vi "Right Execute Motion Profile.vi"(0 "Motor Name":string, 5 "Time Conversion Factor":dbl=0.48, 7 "Linear Conversion Factor":dbl, 9 "Motion Profile Array":dbl[][](array[numeric]), 11 "PIDF Profile Slot Select":u8) -> (4 "Complete":bool, 6 "Motion Profiler Data Out":T1)   [LabVIEW 2016]
uses:
  <vilib>/Rock Robotics/WPI/ThirdParty/CanMotor/TalonSRX/WPI_CANTalonSRX_APIControlMode.ctl
  <vilib>/Rock Robotics/WPI/ThirdParty/CanMotor/TalonSRX/WPI_CANTalonSRX_MotionProfileTrajectoryPt.ctl
  Global Variables/Drive Path Logging Data.vi
panel:
  in  "Motion Profiler Data":T1
  out "Execute Loop Index":i32
  out "Execute Is Last":bool
  out "Mot Prof Active Is Last":bool
  out "Waveform Chart":T2(graph)
  out "Mot Prof Active Is Under Run":bool
  out "Mot Prof Active Is Valid":bool
  out "Mot Prof Buffer Is Full":bool
  out "Mot Prof NextID":i32
  out "Mot Prof Count":i32
  out "Mot Prof Output Enable":i32
  out "Total Points in File":i32
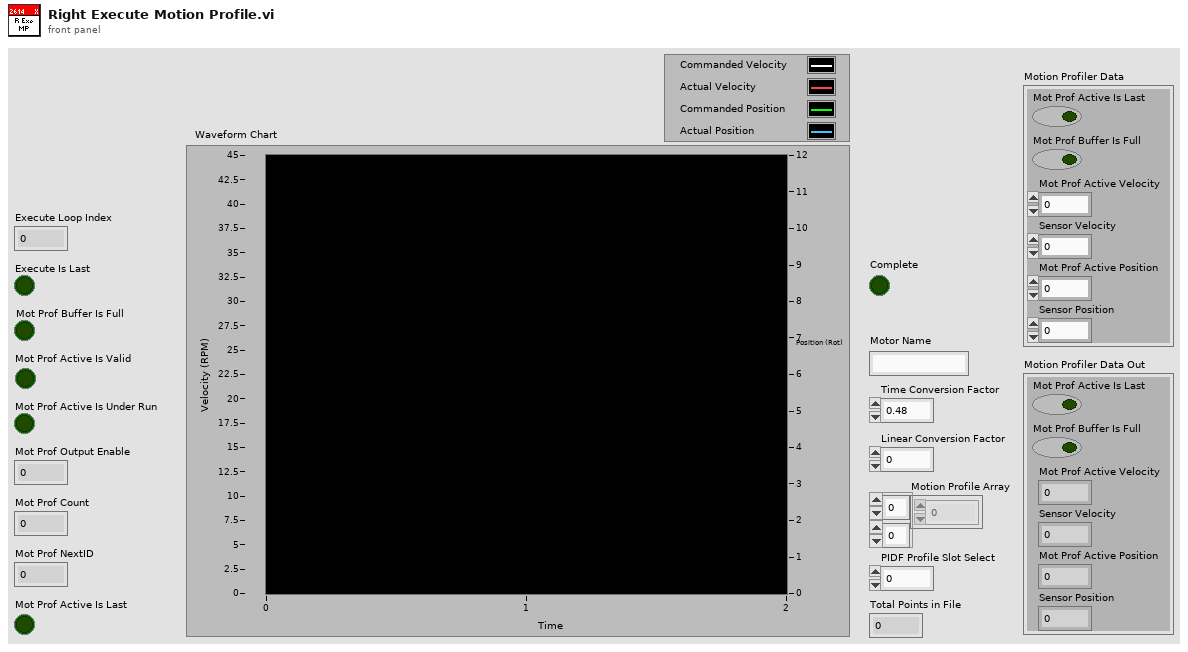
[diagram p1: front panel]
types:
  T1 = cluster{"Mot Prof Active Is Last":bool, "Mot Prof Buffer Is Full":bool, "Mot Prof Active Velocity":dbl, "Sensor Velocity":dbl, "Mot Prof Active Position":dbl, "Sensor Position":dbl}
  T2 = cluster{"Mot Prof Active Velocity":dbl, "Sensor Velocity":dbl, "Mot Prof Active Position":dbl, "Sensor Position":dbl}
  T3 = typedef "WPI_MotorControlDeviceRef.ctl" = cluster{"DeviceStatus":errorcluster, "Type":T4, "PWM":cluster{"PWM Channel":T5, "DeadBand":T6}, "CAN":cluster{"Device Number":u8, "SetOutput VI Ref":variant, "GetOutput VI Ref":variant, "Enable VI Ref":variant, "Disable VI Ref":variant, "Data":variant}, "Invert":bool}
  T4 = typedef "WPI_MotorControlType.ctl" = enum16{"PWM", "CAN"}
  T5 = typedef "FPGA_DIOPWMChannel.ctl" = enum8{"PWM 0", "PWM 1", "PWM 2", "PWM 3", "PWM 4", "PWM 5", "PWM 6", "PWM 7", "PWM 8", "PWM 9", "PWM MXP 0", "PWM MXP 1", "PWM MXP 2", "PWM MXP 3", "PWM MXP 4", "PWM MXP 5", "PWM MXP 6", "PWM MXP 7", "PWM MXP 8", "PWM MXP 9", "Invalid"}
  T6 = typedef "WPI_PWMDeadband.ctl" = cluster{"Name":string, "maxPositivePwm":i32, "minPositivePwm":i32, "centerPwm":i32, "maxNegativePwm":i32, "minNegativePwm":i32, "angularRange":u16}
  T7 = typedef "WPI_CANTalonSRX_APIControlMode.ctl" = enum8{"Percent VBus", "Speed", "Position", "Slave", "Unchanged / Invalid", "Voltage Compensation", "Current", "Motion Profile", "Motion Magic"}
  T8 = typedef "WPI_CANTalonSRX_MotionProfileTrajectoryPt.ctl" = cluster{"Duration Ms":u8, "Velocity":dbl, "Position":dbl, "Profile Slot Select":u8, "Is Last":bool, "Velocity Only":bool, "Zero Position":bool, "Compress Code":u8, "Same Velocity":i32, "Delta Position":i32, "Count":u8}
  T9 = typedef "WPI_CANTalonSRX_GlobalStatus.ctl" = cluster{"Applied Throttle":dbl, "Module Enabled":bool, "CAN Error":errorcluster, "Closed Loop Error":dbl, "Forward Limit Switch Closed":bool, "Reverse Limit Switch Closed":bool, "Sensor Position":dbl, "Sensor Velocity":dbl, "Current":dbl, "Sticky Fault - Over Temp":bool, "Sticky Fault - Under Voltage":bool, "Sticky Fault - Forward Limit":bool, "Sticky Fault - Reverse Limit":bool, "Sticky Fault - Forward Soft Limit":bool, "Sticky Fault - Reverse Soft Limit":bool, "Brake is Enabled":bool, "Encoder Position":dbl, "Encoder Velocity":dbl, "Encoder Index Count":dbl, "Encoder A Pin State":bool, "Encoder B Pin State":bool, "Encoder Index Pin State":bool, "Analog In":dbl, "Analog In Velocity":dbl, "Temperature (C)":dbl, "Battery Voltage":dbl, "Control 5 Is Supported":bool, "Current Profile Slot Select":dbl, "Pos Div 8":bool, "Vel Div 4":bool, "Pulse Width Position":i32, "Pulse Width Velocity":i32, "Pulse Width Rise To Rise (us)":i32, "Pulse Width Rise To Fall (us)":i32, "Mot Prof Active Is Under Run":bool, "Mot Prof Active Has Under Run":bool, "Mot Prof Active Is Last":bool, "Mot Prof Active Velocity Only":bool, "Mot Prof Active Is Valid":bool, "Mot Prof Buffer Is Full":bool, "Mot Prof Active Profile Slot Select":i32, "Mot Prof NextID":i32, "Mot Prof Count":i32, "Mot Prof Active Velocity":dbl, "Mot Prof Active Position":dbl, "Mot Prof Output Enable":i32, "UsageFrame":u32, "Motion Magic Active Trajectory":cluster{"Velocity":dbl, "Position":dbl}}
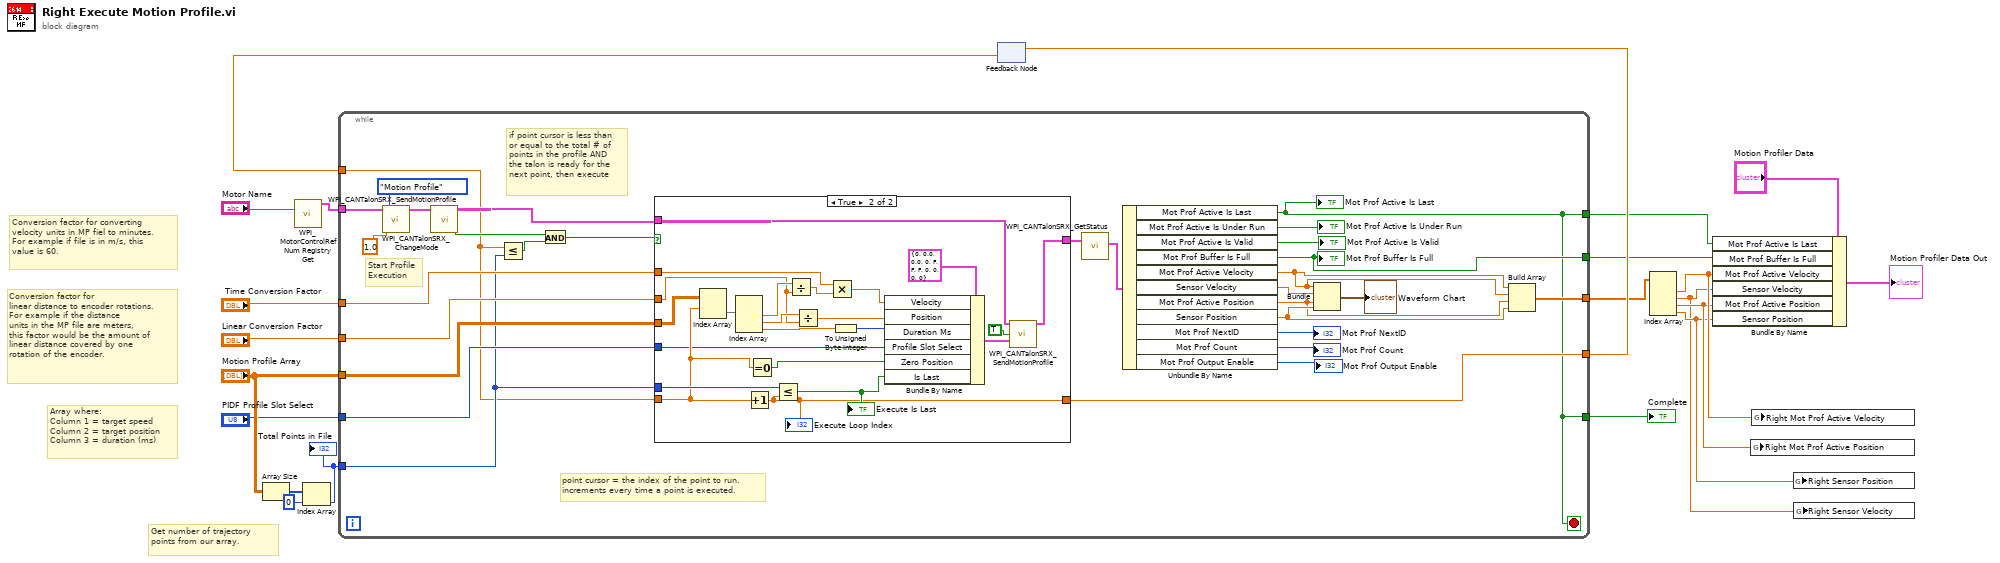
[diagram p0: block diagram]
diagram:
  # "Array where:\nColumn 1 = target speed\nColumn 2 = target position\nColumn 3 = duration (ms)"
  # "Conversion factor for converting \nvelocity units in MP fiel to minutes.\nFor example if file is in m/s, this\nvalue is 60."
  # "Conversion factor for\nlinear distance to encoder rotations.\nFor example if the distance\nunits in the MP file are meters,\nthis factor would be the amount of\nlinear distance covered by one\nrotation of the encoder."
  # "Get number of trajectory points from our array."
  n1 = Array Size(array="Motion Profile Array") -> (size(s)=w21:i32[])
  n2 = call <vilib>:"WPI_MotorControlRefNum Registry Get.vi"("refnum name"="Motor Name") -> ("MotorControlDevRef"=w5:T3)  [unwired: 9 in, 1 out]
  n3 = Index Array(array=w21, index=0) -> (element=w15:i32)
  "Total Points in File" <- w15
  n4 = feedback #1() -> (w13:dbl)  [unwired: 1 in]
  n5 = while {
    tunnel: "Time Conversion Factor" -> [w51]
    tunnel: "Linear Conversion Factor" -> [w50]
    tunnel: "Motion Profile Array" -> [w49]
    tunnel: "PIDF Profile Slot Select" -> [w48]
    tunnel: w15 -> [w47]
    tunnel: w13 -> [w26]
    tunnel: [w27] -> w14
    tunnel: [w25] -> w10
    tunnel: [w23] -> w9
    tunnel: [w24] -> w8
    tunnel: [w23] -> w7
    tunnel: w5 -> [w22]
    stop <- w23 stop-if-true
    # "Start Profile\nExecution"
    # "point cursor = the index of the point to run.\nincrements every time a point is executed."
    # "if point cursor is less than\nor equal to the total # of\npoints in the profile AND\nthe talon is ready for the\nnext point, then execute"
    n6 = call <vilib>:"WPI_CANTalonSRX_ChangeMode.vi"("Output"=1.0, "Control Mode"=WPI_CANTalonSRX_APIControlMode."Motion Profile", "CAN Talon SRX Ref"=w22) -> ("CAN Talon SRX Ref"=w40:T3)  [unwired: 7 in, 1 out]
    n7 = call <vilib>:"WPI_CANTalonSRX_SendMotionProfile.vi"("CAN Talon SRX Ref"=w40) -> ("CAN Talon SRX Ref Out"=w39:T3, "Ready For Next"=w46:bool)  [unwired: 11 in, 2 out]
    n8 = Less Or Equal?(x=w26, y=w47) -> (x <= y?=w44:bool)
    n9 = And(x=w46, y=w44) -> (x .and. y?=w45:bool)
    n10 = case shown="True" w45 {
      tunnel: w39 -> [w52 w70]
      tunnel: w47 -> [_ w69]
      tunnel: w26 -> [w53 w66]
      tunnel: w49 -> [_ w68]
      tunnel: [w53 w65] -> w27
      tunnel: w50 -> [_ w59]
      tunnel: [w52 w57] -> w38
      tunnel: w48 -> [_ w56]
      tunnel: w51 -> [_ w54]
      frame False {
      }
      frame True {
        n11 = Index Array(array=w68, index (row)=w66) -> (element=w67:dbl[])  [unwired: 1 in]
        n12 = Index Array(array=w67) -> (element #1=w63:dbl, element #2=w60:dbl, element #3=w64:dbl)  [unwired: 3 in]
        n13 = Increment(x=w66) -> (x+1=w65:dbl)
        "Execute Loop Index" <- w65
        n14 = Equal To 0?(x=w66) -> (x = 0?=w73:bool)
        n15 = Less Or Equal?(x=w69, y=w65) -> (x <= y?=w72:bool)
        "Execute Is Last" <- w72
        n16 = Divide(x=w63, y=w59) -> (x/y=w62:dbl)
        n17 = Divide(x=w60, y=w59) -> (x/y=w58:dbl)
        n18 = Multiply(x=w54, y=w62) -> (x*y=w61:dbl)
        n19 = To Unsigned Byte Integer(number=w64) -> (unsigned 8bit integer=w55:u8)
        n20 = Bundle By Name(cluster=T8 {"Duration Ms"=0, "Velocity"=0.0, "Position"=0.0, "Profile Slot Select"=0, "Is Last"=FALSE, "Velocity Only"=FALSE, "Zero Position"=FALSE, "Compress Code"=0, "Same Velocity"=0, "Delta Position"=0, "Count"=0} ("New Point"), "Velocity"=w61, "Position"=w58, "Duration Ms"=w55, "Profile Slot Select"=w56, "Zero Position"=w73, "Is Last"=w72) -> (w74:T8)
        n21 = call <vilib>:"WPI_CANTalonSRX_SendMotionProfile.vi"("CAN Talon SRX Ref"=w70, "Push"=TRUE, "New Point"=w74) -> ("CAN Talon SRX Ref Out"=w57:T3)  [unwired: 9 in, 3 out]
      }
    }
    n22 = call <vilib>:"WPI_CANTalonSRX_GetStatus.vi"("CAN Talon SRX Ref"=w38) -> ("Talon SRX Status"=w43:T9)  [unwired: 8 in, 2 out]
    n23 = Unbundle By Name(w43) -> ("Mot Prof Active Is Last"=w23:bool, "Mot Prof Active Is Under Run"=→"Mot Prof Active Is Under Run":bool, "Mot Prof Active Is Valid"=→"Mot Prof Active Is Valid":bool, "Mot Prof Buffer Is Full"=w24:bool, "Mot Prof Active Velocity"=w30:dbl, "Sensor Velocity"=w31:dbl, "Mot Prof Active Position"=w28:dbl, "Sensor Position"=w29:dbl, "Mot Prof NextID"=→"Mot Prof NextID":i32, "Mot Prof Count"=→"Mot Prof Count":i32, "Mot Prof Output Enable"=→"Mot Prof Output Enable":i32)
    "Mot Prof Active Is Last" <- w23
    "Mot Prof Buffer Is Full" <- w24
    n24 = Bundle("Mot Prof Active Velocity"=w30, "Sensor Velocity"=w31, "Mot Prof Active Position"=w28, "Sensor Position"=w29) -> (→"Waveform Chart":T2)  [unwired: 1 in]
    n25 = Build Array(w30, w30, w28, w29) -> (w25:dbl[])
  }
  "Complete" <- w7
  n26 = feedback-in #1(w14) -> ()
  n27 = Index Array(array=w10) -> (element #1=w4:dbl, element #2=w1:dbl, element #3=w3:dbl, element #4=w2:dbl)  [unwired: 4 in]
  n28 = Bundle By Name(cluster="Motion Profiler Data", "Mot Prof Active Is Last"=w9, "Mot Prof Buffer Is Full"=w8, "Mot Prof Active Velocity"=w4, "Sensor Velocity"=w1, "Mot Prof Active Position"=w3, "Sensor Position"=w2) -> (→"Motion Profiler Data Out":T1)
  n29 = global write "Drive Path Logging Data.vi" "Right Mot Prof Active Position"(w3) -> ()
  n30 = global write "Drive Path Logging Data.vi" "Right Mot Prof Active Velocity"(w4) -> ()
  n31 = global write "Drive Path Logging Data.vi" "Right Sensor Position"(w2) -> ()
  n32 = global write "Drive Path Logging Data.vi" "Right Sensor Velocity"(w1) -> ()
